vi "Rename Dependencies.vi"() -> ()   [LabVIEW 2020]
panel:
  in  "reference":refnum<vi>
  in  "delete":bool
  out "Unconverted":path[](array[path])
  out "Original Path":path
  out "File Number":i32
  out "New Path":path
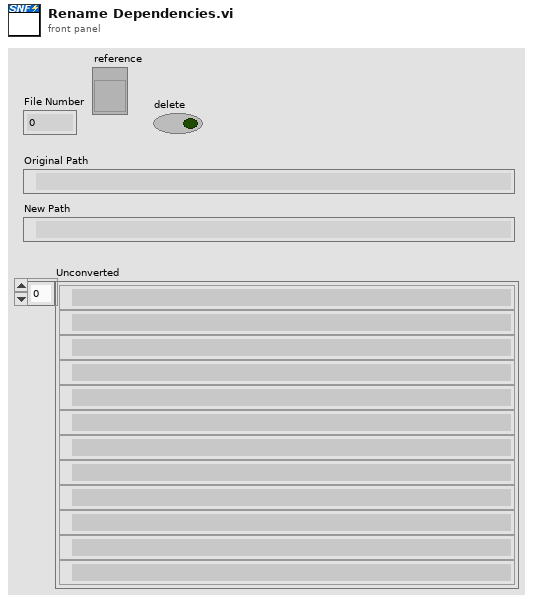
[diagram p1: front panel]
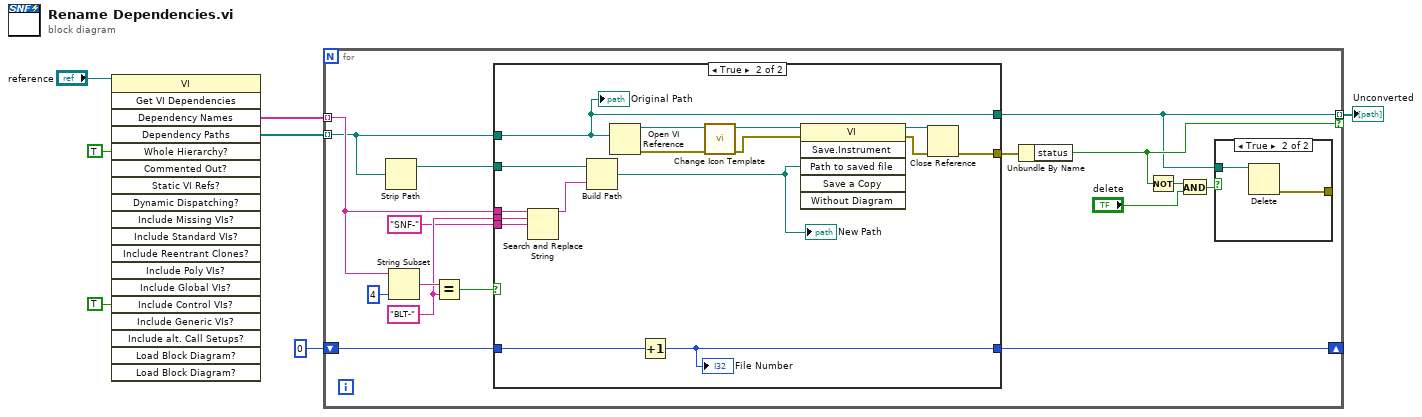
[diagram p0: block diagram]
diagram:
  n1 = invoke class="VI" method="Get VI Dependencies"(reference="reference", "Whole Hierarchy?"=TRUE, "Include Control VIs?"=TRUE) -> ("Dependency Names"=w7:string[], "Dependency Paths"=w6:path[])  [unwired: 16 in, 17 out]
  n2 = for {
    tunnel: w7 -> [w20] mode=indexing
    tunnel: w6 -> [w17] mode=indexing
    shift-right: [w14] -> _
    shift-left: 0 -> [w15]
    tunnel: [w8] -> w3 mode=indexing if=w10
    w19 = "BLT-" ("x")
    n3 = Strip Path(path=w17) -> (stripped path=w21:path)  [unwired: 1 out]
    n4 = String Subset(string=w20, length (rest)=4 ("length (rest)")) -> (substring=w22:string)  [unwired: 1 in]
    n5 = Equal?(x=w22, y=w19) -> (x = y?=w16:bool)
    n6 = case shown="True" w16 {
      tunnel: w21 -> [_ w42]
      tunnel: w20 -> [_ w41]
      tunnel: w19 -> [_ w40]
      tunnel: "SNF-" ("replace string (\"\")") -> [_ w39]
      tunnel: w17 -> [_ w31]
      tunnel: w15 -> [w26 w36]
      tunnel: [w26 w35] -> w14
      tunnel: [_ w32] -> w13
      tunnel: [_ w31] -> w8
      frame False {
      }
      frame True {
        n7 = Search and Replace String(input string=w41, search string=w40, replace string=w39) -> (result string=w38:string)  [unwired: 5 in, 3 out]
        n8 = Build Path(base path=w42, name or relative path=w38) -> (appended path=w37:path)
        "New Path" <- w37
        n9 = Open VI Reference(vi path=w31) -> (vi reference=w30:refnum<vi>, error out=w29:errorcluster)  [unwired: 5 in]
        n10 = Increment(x=w36) -> (x+1=w35:i32)
        "File Number" <- w35
        n11 = call "Change Icon Template.vi"("error in (no error)"=w29, "VI Reference In"=w30) -> ("error out"=w28:errorcluster, "VI Reference Out"=w27:refnum<vi>)  [unwired: 8 in]
        n12 = invoke class="VI" method="Save.Instrument"(reference=w27, error in=w28, "Path to saved file"=w37) -> (reference out=w33:refnum<vi>, error out=w34:errorcluster)  [unwired: 3 in, 4 out]
        n13 = Close Reference(reference=w33, error in (no error)=w34) -> (error out=w32:errorcluster)
        "Original Path" <- w31
      }
    }
    n14 = Unbundle By Name(w13) -> ("status"=w10:bool)
    n15 = Not(x=w10) -> (.not. x?=w11:bool)
    n16 = And(x=w11, y="delete") -> (x .and. y?=w12:bool)
    n17 = case shown="True" w12 {
      tunnel: w8 -> [_ w25]
      tunnel: [_ w24] -> _
      frame False {
      }
      frame True {
        n18 = Delete(path (use dialog)=w25) -> (error out=w24:errorcluster)  [unwired: 4 in, 2 out]
      }
    }
  }
  "Unconverted" <- w3
